vi "ABB make Report browse.vi"(2 "result string":string, 3 "WebBrowser":refnum<k7>(container), 4 "report template folder":path) -> (0 "Report  path":path, 1 "report out":T1)   [LabVIEW 2017]
uses:
  <vilib>/Utility/NIReport.llb/Generate Report Object Reference.ctl
  <vilib>/Utility/NIReport.llb/NI_report.lvclass
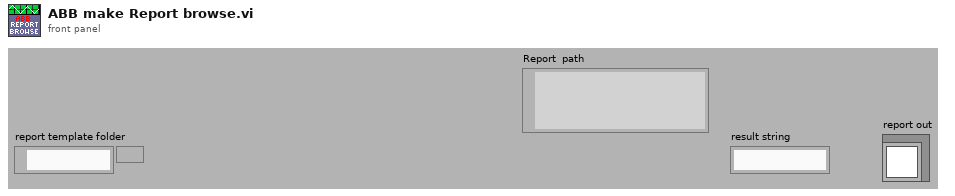
[diagram p1: front panel]
types:
  T1 = typedef "Generate Report Object Reference.ctl" = refnum<class "NI_report.lvclass">
  T2 = cluster{"charset (-1)":i16, "weight (-1)":i16, "name":string, "size":string}
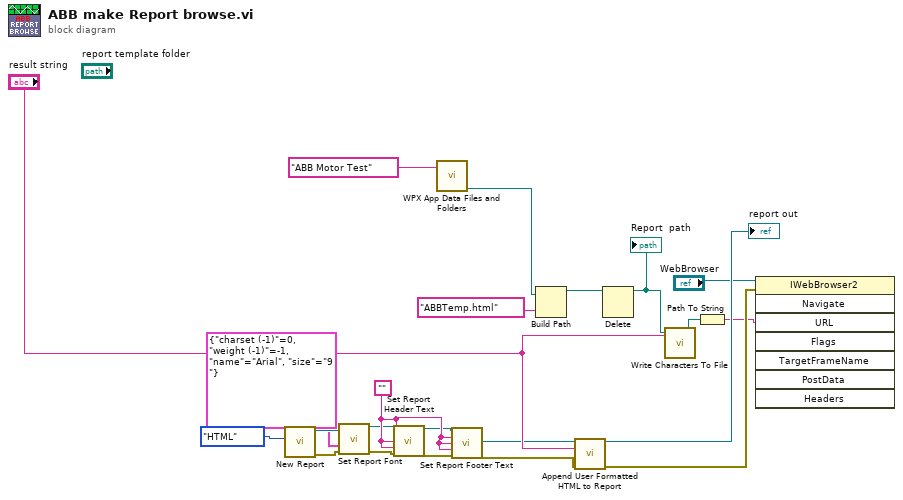
[diagram p0: block diagram]
diagram:
  w21 = ""
  n1 = call <vilib>:"New Report.vi"("report type"=enum16{"Standard Report", "HTML"}."HTML") -> ("report out"=w7:refnum<class "NI_report.lvclass">, "error out"=w6:errorcluster)  [unwired: 13 in]
  n2 = call-dynamic "Set Report Font.vi"("report in"=w7, "font settings"=T2 {"charset (-1)"=0, "weight (-1)"=-1, "name"="Arial", "size"="9 "}, "error in (no error)"=w6) -> ("report out"=w5:refnum<class "NI_report.lvclass">, "error out"=w4:errorcluster)  [unwired: 10 in, 1 out]
  n3 = call-dynamic "Set Report Header Text.vi"("report in"=w5, "left header text"=w21, "center header text"=w21, "right header text"=w21, "error in (no error)"=w4) -> ("report out"=w17:refnum<class "NI_report.lvclass">, "error out"=w18:errorcluster)  [unwired: 9 in]
  n4 = call "WPX App Data Files and Folders.vi"("ApplicationName"="ABB Motor Test") -> ("DataFolder"=w1:path)  [unwired: 7 in, 3 out]
  n5 = call-dynamic "Set Report Footer Text.vi"("report in"=w17, "left footer text"=w21, "center footer text"=w21, "right footer text"=w21, "error in (no error)"=w18) -> ("report out"=w20:refnum<class "NI_report.lvclass">, "error out"=w19:errorcluster)  [unwired: 9 in]
  n6 = Build Path(base path=w1, name or relative path="ABBTemp.html") -> (appended path=w13:path)
  n7 = call-dynamic "Append User Formatted HTML to Report.vi"("report in"=w20, "HTML text"="result string", "error in (no error)"=w19) -> ("report out"=→"report out":refnum<class "NI_report.lvclass">, "error out"=w16:errorcluster)  [unwired: 11 in]
  n8 = Delete(path (use dialog)=w13) -> (deleted path=w14:path)  [unwired: 4 in, 2 out]
  "Report  path" <- w14
  n9 = call <vilib>:"Write Characters To File.vi"("character string"="result string", "file path (dialog if empty)"=w14) -> ("new file path (Not A Path if cancelled)"=w10:path)  [unwired: 3 in]
  n10 = Path To String(path=w10) -> (string=w11:string)
  n11 = invoke class="IWebBrowser2" method="Navigate"(reference="WebBrowser", error in=w16, "URL"=w11) -> ()  [unwired: 5 in, 8 out]
